vi "Process Live Data Q Mov.vi"(8 "error in (no error)":errorcluster, 10 "Live Data Q Elements":cluster{"NI Data Waveforms":waveform(dbl)[]}[](array[cluster]), 11 "NI Force Task in":refnum<class "NI Force Task.lvclass">) -> (0 "error out":errorcluster, 3 "NI Force Task out":refnum<class "NI Force Task.lvclass">)   [LabVIEW 2020, in "NI Force Task.lvlib" / "NI Force Task.lvclass"]
uses:
  NI Force Task.lvclass
  NI Force Task.lvclass/NI Force Task.ctl
  <vilib>/Analysis/baseanly.llb/Mean (DBL).vi
  <vilib>/Analysis/NI_AALBase.lvlib
  Task Viewer Messages/Receive Q Msg/Receive Q Msg.lvclass
  Lissajous Viewer Messages/Update graph Msg/Update graph Msg.lvclass
panel:
  out "error out 2":errorcluster
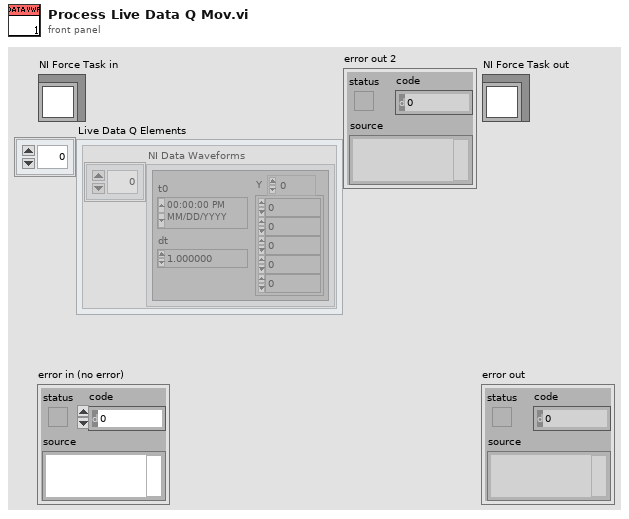
[diagram p1: front panel]
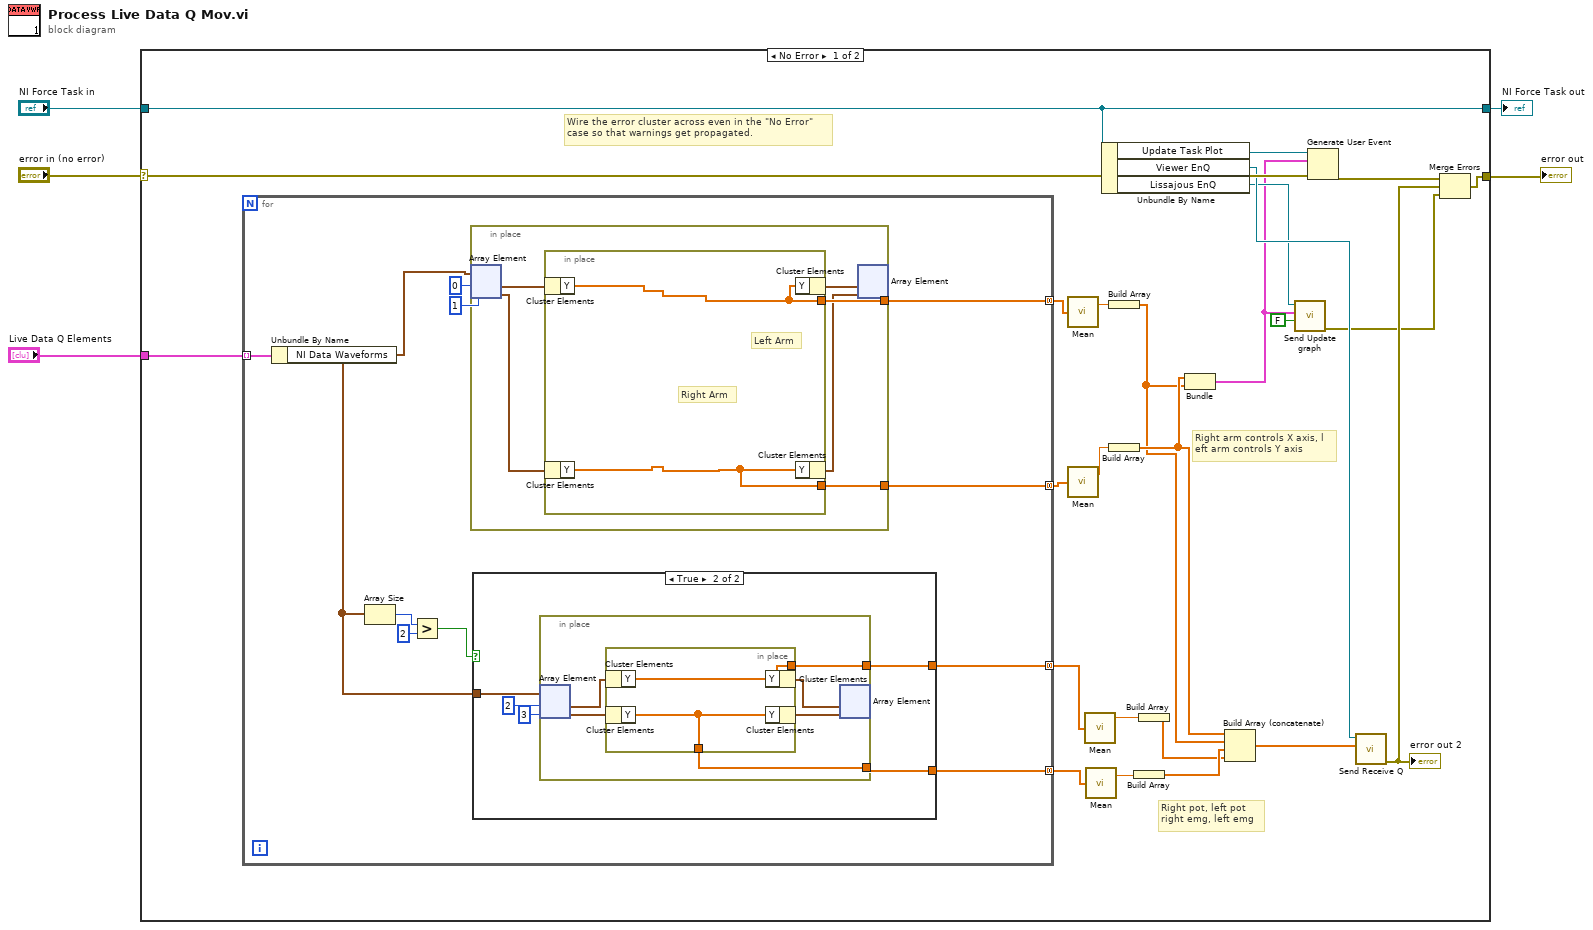
[diagram p0: block diagram]
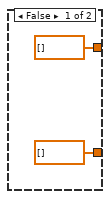
[diagram p2: hidden frame]
diagram:
  n1 = case shown="No Error" "error in (no error)" {
    selector: "error in (no error)" -> [w23 w65]
    tunnel: [w30 w66] -> w3
    tunnel: "NI Force Task in" -> [w30 w66]
    tunnel: "Live Data Q Elements" -> [w29 _]
    tunnel: [w15 w65] -> w1
    frame No Error {
      # "Right pot, left pot\nright emg, left emg"
      # "Right arm controls X axis, l\neft arm controls Y axis"
      # "Wire the error cluster across even in the \"No Error\"\ncase so that warnings get propagated."
      n2 = for {
        tunnel: w29 -> [w41] mode=indexing
        tunnel: [w39] -> w26 mode=concatenating
        tunnel: [w38] -> w25 mode=concatenating
        tunnel: [w32] -> w22 mode=concatenating
        tunnel: [w31] -> w21 mode=concatenating
        n3 = Unbundle By Name(w41) -> ("NI Data Waveforms"=w33:waveform(dbl)[])
        n4 = Array Size(array=w33) -> (size(s)=w36:i32)
        n5 = Greater?(x=w36, y=2) -> (0:w34:bool)
        n6 = in-place {
          in-place-border: [w60] -> w39
          in-place-border: [w59] -> w38
          n7 = in-place-array #1(w33, 0, 1) -> (w62:waveform(dbl), w58:waveform(dbl))
          n8 = in-place {
            in-place-border: [w64] -> w60
            in-place-border: [w63] -> w59
            # "Right Arm"
            # "Left Arm"
            n9 = in-place-cluster #2(w62) -> ("Y"=w64:dbl[])
            n10 = in-place-cluster #3(w58) -> ("Y"=w63:dbl[])
            n11 = in-place-cluster #2("Y"=w64) -> (w61:waveform(dbl))
            n12 = in-place-cluster #3("Y"=w63) -> (w57:waveform(dbl))
          }
          n13 = in-place-array #1(w61, w57) -> ()  [unwired: 3 out]
        }
        n14 = case shown="True" w34 {
          tunnel: w33 -> [_ w48]
          tunnel: [dbl[] [] ("Y") w45] -> w32
          tunnel: [dbl[] [] ("Y") w44] -> w31
          frame False {
          }
          frame True {
            n15 = in-place {
              in-place-border: [w50] -> w45
              in-place-border: [w49] -> w44
              n16 = in-place-array #4(w48, 2, 3) -> (w54:waveform(dbl), w53:waveform(dbl))
              n17 = in-place {
                in-place-border: [w56] -> w50
                in-place-border: [w55] -> w49
                n18 = in-place-cluster #5(w54) -> ("Y"=w56:dbl[])
                n19 = in-place-cluster #6(w53) -> ("Y"=w55:dbl[])
                n20 = in-place-cluster #5("Y"=w56) -> (w52:waveform(dbl))
                n21 = in-place-cluster #6("Y"=w55) -> (w51:waveform(dbl))
              }
              n22 = in-place-array #4(w52, w51) -> ()  [unwired: 3 out]
            }
          }
        }
      }
      n23 = call-poly <vilib>:"Mean.vi"("X"=w26) -> ("mean"=w28:dbl)  [unwired: 1 out]
      n24 = call-poly <vilib>:"Mean.vi"("X"=w25) -> ("mean"=w27:dbl)  [unwired: 1 out]
      n25 = call-poly <vilib>:"Mean.vi"("X"=w22) -> ("mean"=w19:dbl)  [unwired: 1 out]
      n26 = call-poly <vilib>:"Mean.vi"("X"=w21) -> ("mean"=w20:dbl)  [unwired: 1 out]
      n27 = Unbundle By Name(w30) -> ("Update Task Plot"=w24:refnum<user-event>, "Viewer EnQ"=w16:refnum<class "Message Enqueuer.lvclass">, "Lissajous EnQ"=w9:refnum<class "Message Enqueuer.lvclass">)
      n28 = Build Array(w28) -> (w10:dbl[])
      n29 = Build Array(w27) -> (w11:dbl[])
      n30 = Build Array(w20) -> (w18:dbl[])
      n31 = Build Array(w19) -> (w17:dbl[])
      n32 = Bundle(w11, w10) -> (w8:cluster{dbl[], dbl[]})  [unwired: 1 in]
      n33 = Build Array (concatenate)(w11, w10, w18, w17) -> (w12:dbl[])
      n34 = call "Send Update graph.vi"("Template?"=FALSE, "Data"=w8, "Message Enqueuer in"=w9) -> ("error out"=w6:errorcluster)  [unwired: 7 in, 1 out]
      n35 = Generate User Event(user event=w24, event data cluster=w8, error in=w23) -> (error out=w14:errorcluster)  [unwired: 1 in, 1 out]
      n36 = call "Send Receive Q.vi"("Disp Data"=w12, "Message Enqueuer in"=w16) -> ("error out"=w13:errorcluster)  [unwired: 8 in, 1 out]
      "error out 2" <- w13
      n37 = Merge Errors(w14, w13, w6) -> (w15:errorcluster)
    }
    frame Error {
    }
  }
  "error out" <- w1
  "NI Force Task out" <- w3
